vi "test12.3-AsyncMessageWithoutReply_Event.vi"(8 "error in (no error)":errorcluster, 11 "TestCase in":refnum<class "testcase-CSMGlobalLog.lvclass">) -> (0 "error out":errorcluster, 3 "TestCase out":refnum<class "testcase-CSMGlobalLog.lvclass">)   [LabVIEW 2017, in "testcase-CSMGlobalLog.lvclass"]
uses:
  testcase-CSMGlobalLog.lvclass
  testcase-CSMGlobalLog.lvclass/testcase-CSMGlobalLog.ctl
  src/user.lib/_NEVSTOP/Communicable State Machine(CSM)/_Support/Typedef/_CSM_GlobalLog_MSG.ctl
  src/user.lib/_NEVSTOP/Communicable State Machine(CSM)/_Support/Typedef/_CSM_Response Source Message.ctl
  src/user.lib/_NEVSTOP/Communicable State Machine(CSM)/_Support/Typedef/_CSM_GlobalLog_MSG_TYPE.ctl
  c0dc643a-0362-49fc-99f4-5251266ba5a0.vi
  src/user.lib/_NEVSTOP/Communicable State Machine(CSM)/_Support/GlobalEvent/GEvt-Generate with Rule Check.vi
  src/user.lib/_NEVSTOP/Communicable State Machine(CSM)/AdvanceAPI/CSM - Convert Error to Argument.vi
  src/user.lib/_NEVSTOP/Communicable State Machine(CSM)/AdvanceAPI/CSM - Make String Arguments Safe.vi
  src/user.lib/_NEVSTOP/Communicable State Machine(CSM)/AdvanceAPI/CSM - Keywords.vi
  src/user.lib/_NEVSTOP/Communicable State Machine(CSM)/_Support/GlobalEvent/Cache-GEvt Refs.vi
  src/user.lib/_NEVSTOP/Communicable State Machine(CSM)/_Support/GlobalEvent/LogFilter/LogFilter - Check.vi
  src/user.lib/_NEVSTOP/Communicable State Machine(CSM)/_Support/GlobalEvent/LogFilter/LogFilter.lvclass
  <vilib>/addons/_JKI Toolkits/VI Tester/TestCase.llb/TestCase.lvclass
  src/user.lib/_NEVSTOP/Communicable State Machine(CSM)/Communicable State Machine.lvlib
  CSM/CSM-Testcase.lvlib
  C:/Program Files (x86)/National Instruments/LabVIEW 2017/vi.lib/addons/_JKI Toolkits/VI Tester/TestCase.llb/TestCase.lvclass
panel:
  out "String cache each loop":string
  out "LoopCount":i32
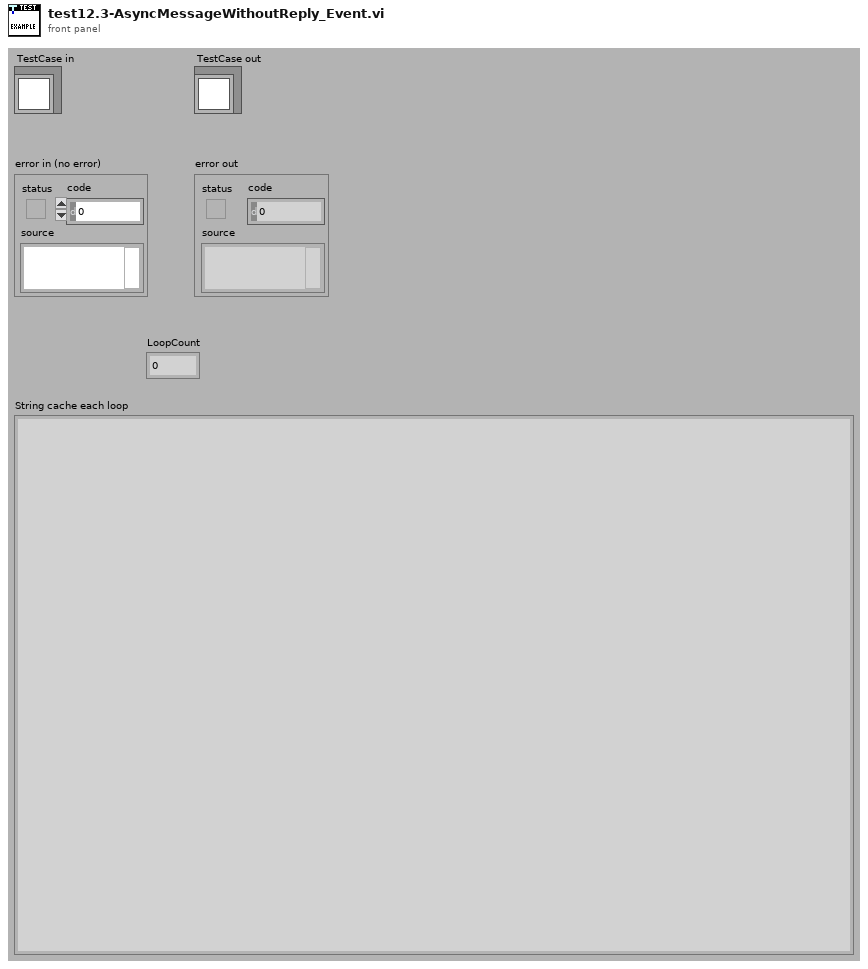
[diagram p1: front panel]
types:
  T1 = typedef "Communicable State Machine.lvlib/_CSM_GlobalLog_MSG.ctl" = cluster{"Name (\"\" to Use UUID)":string, "Current State":string, "Arguments":string, "Source Message":T2, "Source Module":string, "Complete(T)/Start(F)":bool, "LogType":T3, "Time Stamp":timestamp}
  T2 = typedef "Communicable State Machine.lvlib/_CSM_Response Source Message.ctl" = cluster{"‘State":string, "’Arguments":string, "’Error":errorcluster}
  T3 = typedef "Communicable State Machine.lvlib/_CSM_GlobalLog_MSG_TYPE.ctl" = enum16{"User Log", "State Change", "Status", "Interrupt", "Register", "Unregister", "Error Log", "Module Created", "Module Destroyed", "Async Message", "No-Rep Async Message", "Sync Message"}
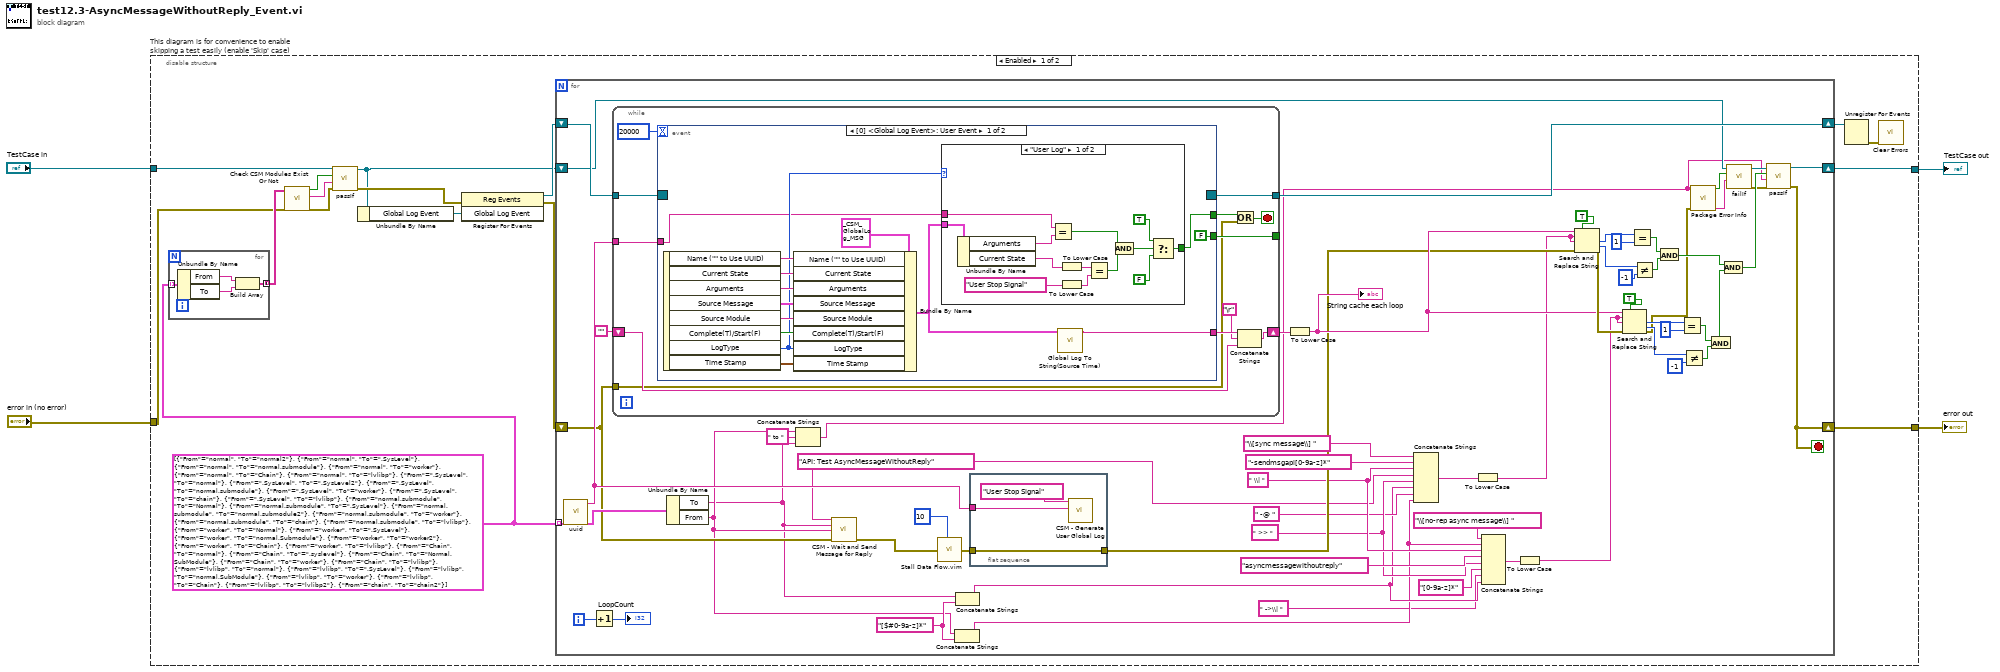
[diagram p0: block diagram]
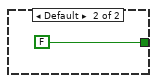
[diagram p2: hidden frame]
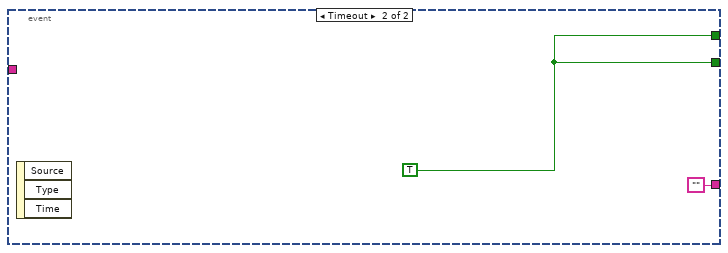
[diagram p3: hidden frame]
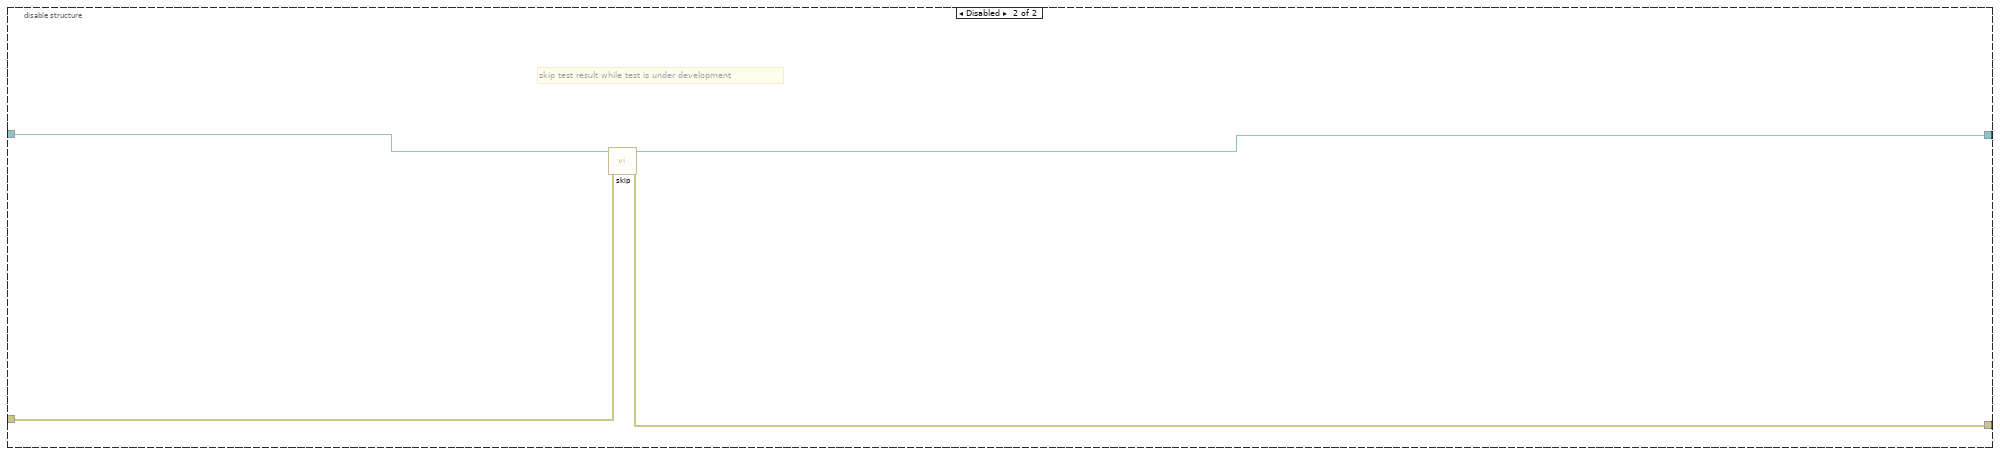
[diagram p4: hidden frame]
diagram:
  n1 = disable-structure "This diagram is for convenience to enable skipping a test easily (enable 'Skip' case)" shown="Enabled" {
    disable-tunnel: "TestCase in" -> [w7 w134]
    disable-tunnel: [w16 w132] -> w1
    disable-tunnel: [w15 w133] -> w3
    disable-tunnel: "error in (no error)" -> [w9 w131]
    frame Enabled {
      w10 = cluster{"From":string, "To":string}[] [{"From"="normal", "To"="normal2"}, {"From"="normal", "To"=".SysLevel"}, {"From"="normal", "To"="normal.submodule"}, {"From"="normal", "To"="worker"}, {"From"="normal", "To"="Chain"}, {"From"="normal", "To"="lvlibp"}, {"From"=".SysLevel", "To"="normal"}, {"From"=".SysLevel", "To"=".SysLevel2"}, {"From"=".SysLevel", "To"="normal.submodule"}, {"From"=".SysLevel", "To"="worker"}, {"From"=".SysLevel", "To"="chain"}, {"From"=".SysLevel", "To"="lvlibp"}, {"From"="normal.submodule", "To"="Normal"}, {"From"="normal.submodule", "To"=".SysLevel"}, {"From"="normal.submodule", "To"="normal.submodule2"}, {"From"="normal.submodule", "To"="worker"}, {"From"="normal.submodule", "To"="chain"}, {"From"="normal.submodule", "To"="lvlibp"}, {"From"="worker", "To"="Normal"}, {"From"="worker", "To"=".SysLevel"}, {"From"="worker", "To"="normal.Submodule"}, {"From"="worker", "To"="worker2"}, {"From"="worker", "To"="Chain"}, {"From"="worker", "To"="lvlibp"}, {"From"="Chain", "To"="normal"}, {"From"="Chain", "To"=".syslevel"}, {"From"="Chain", "To"="Normal.SubModule"}, {"From"="Chain", "To"="worker"}, {"From"="Chain", "To"="lvlibp"}, {"From"="lvlibp", "To"="normal"}, {"From"="lvlibp", "To"=".SysLevel"}, {"From"="lvlibp", "To"="normal.SubModule"}, {"From"="lvlibp", "To"="worker"}, {"From"="lvlibp", "To"="Chain"}, {"From"="lvlibp", "To"="lvlibp2"}, {"From"="chain", "To"="chain2"}]
      n2 = for {
        tunnel: w10 -> [w24] mode=indexing
        tunnel: [w21] -> w13 mode=concatenating
        n3 = Unbundle By Name(w24) -> ("From"=w23:string, "To"=w22:string)
        n4 = Build Array(w23, w22) -> (w21:string[])
      }
      n5 = call "Check CSM Modules Exist Or Not.vi"("error in"=w9, "CSM names in"=w13) -> ("error out"=w11:errorcluster, "Debug string"=w12:string, "All Modules Exist?"=w14:bool)  [unwired: 7 in]
      n6 = call-dynamic "passIf.vi"("error in (no error)"=w11, "message (\"\")"=w12, "pass"=w14, "TestCase in"=w7) -> ("error out"=w8:errorcluster, "TestCase out"=w6:refnum<class "testcase-CSMGlobalLog.lvclass">)  [unwired: 6 in]
      n7 = Unbundle By Name(w6) -> ("Global Log Event"=w20:refnum<user-event>)
      n8 = register-events(error in=w8, w20) -> (reference out=w19:refnum<event-registration>, error out=w17:errorcluster)  [unwired: 1 in]
      n9 = for {
        shift-right: [w84] -> w18
        shift-left: w19 -> [w85]
        shift-right: [w81] -> w15
        shift-left: w17 -> [w35]
        tunnel: w10 -> [w62] mode=indexing
        shift-right: [w83] -> w16
        shift-left: w6 -> [w33]
        i -> [w59]
        stop <- w81 stop-if-true
        w40 = "[$#0-9a-z]*" ("string")
        w48 = " >> "
        w50 = " \\| "
        w43 = "API: Test AsyncMessageWithoutReply" ("State")
        n10 = call "uuid.vi"() -> ("UUID"=w60:string)  [unwired: 11 in]
        n11 = Increment(x=w59) -> (x+1=→"LoopCount":i32)
        n12 = while {
          tunnel: w85 -> [w100]
          tunnel: [w99] -> w84
          shift-right: [w91] -> w53
          shift-left: "" -> [w94]
          tunnel: w60 -> [w96]
          tunnel: [w95] -> _
          tunnel: w35 -> [w89]
          stop <- w90 stop-if-true
          n13 = event shown="[0] <Global Log Event>: User Event" {
            selector: w100 -> [_ _]
            dyn-events: [_ _] -> w99
            timeout: 20000 -> [_ _]
            tunnel: [w101 ""] -> w93
            tunnel: [w103 w130] -> w98
            tunnel: w96 -> [w104 _]
            tunnel: [FALSE ("Stop") w130] -> w95
            event User Event {
              n14 = event-data() -> ("Name (\"\" to Use UUID)"=w113:string, "Current State"=w112:string, "Arguments"=w111:string, "Source Message"=w110:T2, "Source Module"=w109:string, "Complete(T)/Start(F)"=w108:bool, "LogType"=w105:T3, "Time Stamp"=w107:timestamp)  [unwired: 1 in]
              n15 = Bundle By Name(cluster=T1 {"Name (\"\" to Use UUID)"="", "Current State"="", "Arguments"="", "Source Message"={"‘State"="", "’Arguments"="", "’Error"={"status"=FALSE, "code"=0, "source"=""}}, "Source Module"="", "Complete(T)/Start(F)"=FALSE, "LogType"=enum."State Change", "Time Stamp"=timestamp(0 s since 1904-01-01)} ("Cross CSM Data"), "Name (\"\" to Use UUID)"=w113, "Current State"=w112, "Arguments"=w111, "Source Message"=w110, "Source Module"=w109, "Complete(T)/Start(F)"=w108, "LogType"=w105, "Time Stamp"=w107) -> (w102:T1)
              n16 = case shown="\"User Log\"" w105 {
                tunnel: w102 -> [w127 _]
                tunnel: w104 -> [w126 _]
                tunnel: [w115 FALSE] -> w103
                frame "User Log" {
                  n17 = Unbundle By Name(w127) -> ("Arguments"=w125:string, "Current State"=w124:string)
                  n18 = Equal?(x=w126, y=w125) -> (x = y?=w119:bool)
                  n19 = To Lower Case(string=w124) -> (all lower case string=w123:string)
                  n20 = To Lower Case(string="User Stop Signal" ("Log")) -> (all lower case string=w121:string)
                  n21 = Equal?(x=w123, y=w121) -> (x = y?=w120:bool)
                  n22 = And(x=w119, y=w120) -> (x .and. y?=w118:bool)
                  n23 = Select(t=TRUE, s=w118, f=FALSE) -> (s? t:f=w115:bool)
                }
                frame Default {
                }
              }
              n24 = call "Global Log To String(Source Time).vi"("Log"=w102) -> ("Log String"=w101:string)  [unwired: 9 in]
            }
            event Timeout {
              w130 = TRUE ("Stop")
              n25 = event-data() -> ()  [unwired: 1 in, 3 out]
            }
          }
          n26 = Or(x=w98, y=w89) -> (x .or. y?=w90:bool)
          n27 = Concatenate Strings(w93, "\r", w94) -> (w91:string)
        }
        n28 = Unbundle By Name(w62) -> ("To"=w27:string, "From"=w28:string)
        n29 = Concatenate Strings(w28, " to " ("string"), w27) -> (w25:string)
        n30 = call "CSM - Wait and Send Message for Reply.vi"("State"=w43, "Arguments (\"\")"=w27, "Target Module"=w28, "Error In (No Error)"=w35) -> ("error out"=w56:errorcluster)  [unwired: 8 in, 3 out]
        n31 = call "Stall Data Flow.vim"("value in"=w56, "milliseconds to wait"=u32 10) -> ("value out"=w61:errorcluster)  [unwired: 1 out]
        n32 = Concatenate Strings(w28, w40) -> (w38:string)
        n33 = Concatenate Strings(w27, w40) -> (w39:string)
        n34 = flat-sequence {
          tunnel: w60 -> [w87]
          tunnel: w61 -> [w86]
          tunnel: [w86] -> w54
          frame #0 {
            n35 = call "CSM - Generate User Global Log.vi"("Arguments"=w87, "Log"="User Stop Signal") -> ()  [unwired: 9 in, 1 out]
          }
        }
        n36 = To Lower Case(string=w53) -> (all lower case string=w55:string)
        "String cache each loop" <- w55
        n37 = Concatenate Strings("\\[sync message\\] ", "-sendmsgapi[0-9a-z]*", w50, w43, w48, w39, " -@ ", w38) -> (w45:string)
        n38 = To Lower Case(string=w45) -> (all lower case string=w42:string)
        n39 = Concatenate Strings("\\[no-rep async message\\] " ("string"), w38, w50, "asyncmessagewithoutreply", w48, "[0-9a-z]*", " ->\\| ", w39) -> (w44:string)
        n40 = To Lower Case(string=w44) -> (all lower case string=w41:string)
        n41 = Search and Replace String(replace all?=TRUE ("replace all? (F)"), input string=w55, search string=w42, replace string=w42, error in=w54) -> (number of replacements=w70:i32, offset past replacement=w71:i32, error out=w78:errorcluster)  [unwired: 3 in, 1 out]
        n42 = Search and Replace String(replace all?=TRUE ("replace all? (F)"), input string=w55, search string=w41, replace string=w41, error in=w78) -> (number of replacements=w77:i32, offset past replacement=w76:i32, error out=w29:errorcluster)  [unwired: 3 in, 1 out]
        n43 = Equal?(x=w70, y=1) -> (x = y?=w72:bool)
        n44 = Not Equal?(x=w71, y=-1) -> (x != y?=w73:bool)
        n45 = And(x=w72, y=w73) -> (x .and. y?=w80:bool)
        n46 = Equal?(x=w77, y=1) -> (x = y?=w75:bool)
        n47 = Not Equal?(x=w76, y=-1) -> (x != y?=w74:bool)
        n48 = call "Package Error Info.vi"("error in"=w29, "String in"=w25) -> ("packed error info out"=w30:string, "error status"=w34:bool)  [unwired: 8 in]
        n49 = And(x=w75, y=w74) -> (x .and. y?=w79:bool)
        n50 = And(x=w80, y=w79) -> (x .and. y?=w58:bool)
        n51 = call-dynamic "failIf.vi"("message (\"\")"=w30, "fail"=w34, "TestCase in"=w33) -> ("error out"=w31:errorcluster, "TestCase out"=w32:refnum<class "testcase-CSMGlobalLog.lvclass">)  [unwired: 7 in]
        n52 = call-dynamic "passIf.vi"("error in (no error)"=w31, "message (\"\")"=w25, "pass"=w58, "TestCase in"=w32) -> ("error out"=w81:errorcluster, "TestCase out"=w83:refnum<class "testcase-CSMGlobalLog.lvclass">)  [unwired: 6 in]
      }
      n53 = Unregister For Events(event registration refnum=w18) -> (error out=w5:errorcluster)  [unwired: 1 in]
      n54 = call <vilib>:"Clear Errors.vi"("error in (no error)"=w5) -> ()  [unwired: 5 in, 2 out]
    }
    frame Disabled {
      # "skip test result while test is under development"
      n55 = call <vilib>:"skip.vi"("error in (no error)"=w131, "TestCase in"=w134) -> ("error out"=w133:errorcluster, "TestCase out"=w132:refnum<class "testcase-CSMGlobalLog.lvclass">)  [unwired: 8 in]
    }
  }
  "error out" <- w3
  "TestCase out" <- w1
